vi "SetStimulusParametersGUI.vi"(8 "error in (no error)":errorcluster, 11 "StimulusObject in":refnum<class "StimulusObject.lvclass">) -> (0 "error out":errorcluster, 2 "Parameter Array Out":sgl[](array[numeric]), 3 "StimulusObject out":refnum<class "StimulusObject.lvclass">)   [LabVIEW 2019, in "StimulusObject.lvclass"]
uses:
  StimulusObject.lvclass
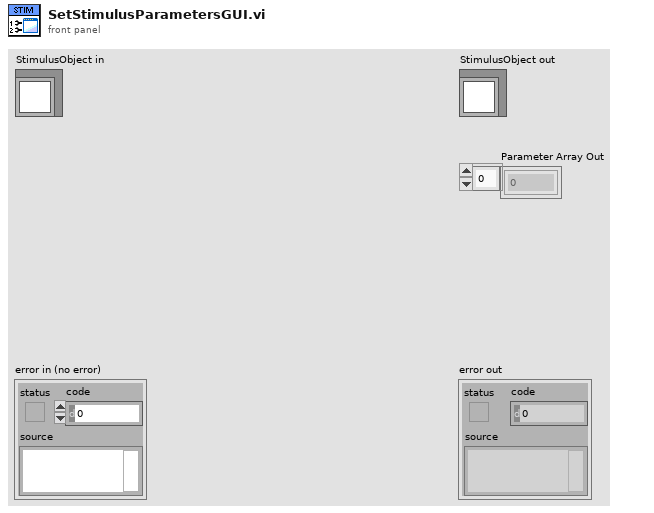
[diagram p1: front panel]
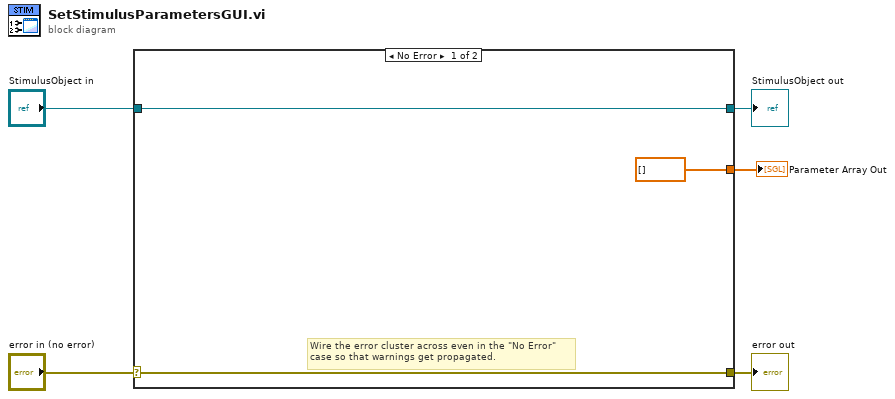
[diagram p0: block diagram]
diagram:
  n1 = case shown="No Error" "error in (no error)" {
    selector: "error in (no error)" -> [w7 w10]
    tunnel: [w7 w10] -> w4
    tunnel: [w8 w9] -> w2
    tunnel: "StimulusObject in" -> [w8 w9]
    tunnel: [sgl[] [] ("Parameter Array") _] -> w1
    frame No Error {
      # "Wire the error cluster across even in the \"No Error\"\ncase so that warnings get propagated."
    }
    frame Error {
    }
  }
  "error out" <- w4
  "StimulusObject out" <- w2
  "Parameter Array Out" <- w1
